vi "ptp.vi"() -> ()   [LabVIEW 2017]
uses:
  <vilib>/MediaMongrels Ltd/WebSockets/WebSockets/WebSocket Client/WebSocket Client.lvclass
panel:
  out "jumpHeight":dbl
  out "zLimit":dbl
  out "acceleration":dbl[](array[numeric])
  out "velocity":dbl[](array[numeric])
  in  "id":i32
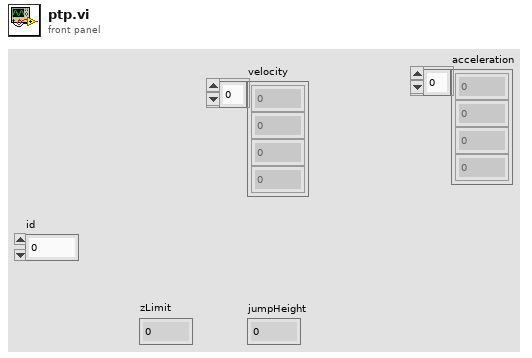
[diagram p1: front panel]
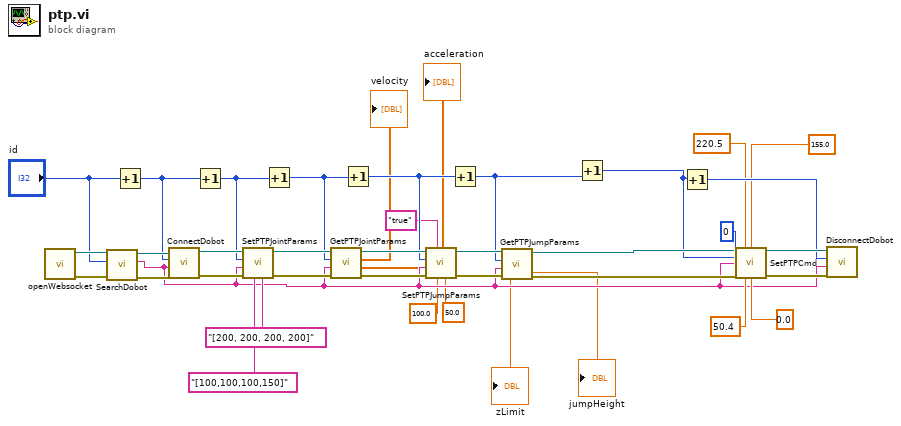
[diagram p0: block diagram]
diagram:
  n1 = call <vilib>:"openWebsocket.vi"() -> ("error out"=w39:errorcluster, "WebSocket Client out"=w37:refnum<class "WebSocket Client.lvclass">)  [unwired: 10 in]
  n2 = call <vilib>:"SearchDobot.vi"("error in (no error)"=w39, "id"="id", "WebSocket in"=w37) -> ("error out"=w38:errorcluster, "portName"=w8:string, "WebSocket out"=w36:refnum<class "WebSocket Client.lvclass">)  [unwired: 6 in]
  n3 = Increment(x="id") -> (x+1=w33:i32)
  n4 = call <vilib>:"ConnectDobot.vi"("error in (no error)"=w38, "portName"=w8, "id"=w33, "WebSocket in"=w36) -> ("error out"=w29:errorcluster, "WebSocket out"=w30:refnum<class "WebSocket Client.lvclass">)  [unwired: 5 in, 1 out]
  n5 = Increment(x=w33) -> (x+1=w28:i32)
  n6 = call <vilib>:"SetPTPJointParams.vi"("acceleration"="[200, 200, 200, 200]", "velocity"="[100,100,100,150]", "error in (no error)"=w29, "portName"=w8, "id"=w28, "WebSocket in"=w30) -> ("error out"=w24:errorcluster, "WebSocket out"=w25:refnum<class "WebSocket Client.lvclass">)  [unwired: 3 in, 1 out]
  n7 = Increment(x=w28) -> (x+1=w23:i32)
  n8 = call <vilib>:"GetPTPJointParams.vi"("error in (no error)"=w24, "portName"=w8, "id"=w23, "WebSocket in"=w25) -> ("error out"=w14:errorcluster, "acceleration"=→"acceleration":dbl[], "velocity"=→"velocity":dbl[], "WebSocket out"=w17:refnum<class "WebSocket Client.lvclass">)  [unwired: 4 in]
  n9 = Increment(x=w23) -> (x+1=w10:i32)
  n10 = call <vilib>:"SetPTPJumpParams.vi"("jumpHeight"=50.0, "zLimit"=100.0, "isUsingZLimit"="true", "error in (no error)"=w14, "portName"=w8, "id"=w10, "WebSocket in"=w17) -> ("error out"=w13:errorcluster, "WebSocket out"=w16:refnum<class "WebSocket Client.lvclass">)  [unwired: 2 in, 1 out]
  n11 = Increment(x=w10) -> (x+1=w9:i32)
  n12 = call <vilib>:"GetPTPJumpParams.vi"("error in (no error)"=w13, "portName"=w8, "id"=w9, "WebSocket in"=w16) -> ("error out"=w12:errorcluster, "WebSocket out"=w15:refnum<class "WebSocket Client.lvclass">, "jumpHeight"=→"jumpHeight":dbl, "zLimit"=→"zLimit":dbl)  [unwired: 3 in, 1 out]
  n13 = Increment(x=w9) -> (x+1=w11:i32)
  n14 = Increment(x=w11) -> (x+1=w32:i32)
  n15 = call <vilib>:"SetPTPCmd.vi"("WebSocket in"=w15, "x"=220.5, "y"=155.0, "id"=w11, "portName"=w8, "ptpMode"=0, "error in (no error)"=w12, "z"=50.4, "r"=0.0) -> ("WebSocket out"=w35:refnum<class "WebSocket Client.lvclass">, "error out"=w34:errorcluster)  [unwired: 4 in, 1 out]
  n16 = call <vilib>:"DisconnectDobot.vi"("error in (no error)"=w34, "portName"=w8, "id"=w32, "WebSocket in"=w35) -> ()  [unwired: 5 in, 3 out]
